vi "Find Optimal IRF Tail Slope.vi"(11 "Slope Array":dbl[](array[numeric])) -> (1 "Optimal Index":i32, 3 "Optimal Slope":dbl)   [LabVIEW 2021, in "Fits.lvlib"]
doc: "Find minimal absolute slope for the optimal IRF extraction algorithm."
uses:
  Fits.lvlib
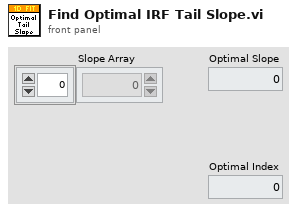
[diagram p1: front panel]
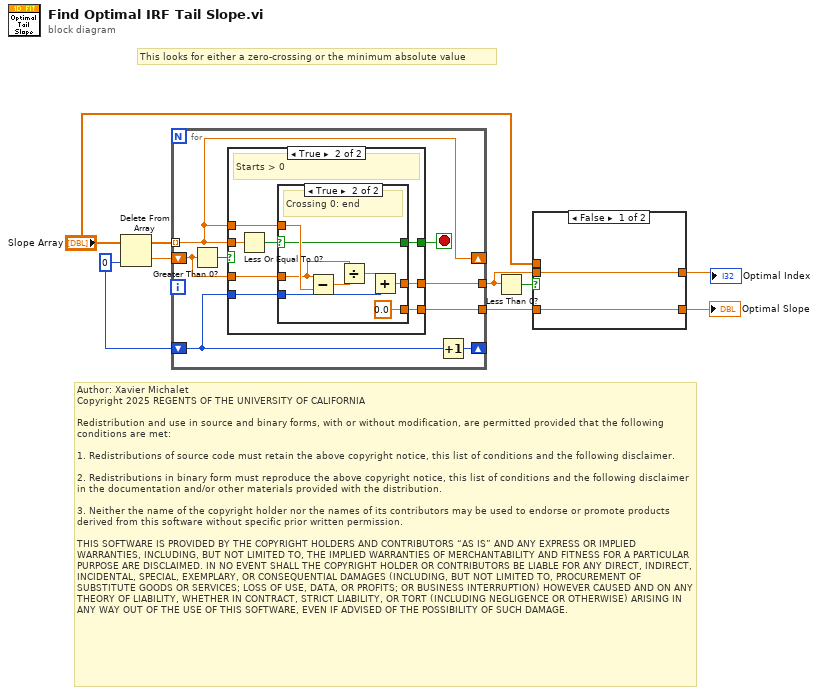
[diagram p0: block diagram]
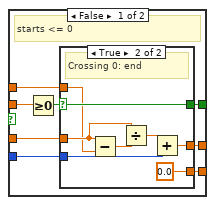
[diagram p2: hidden frame]
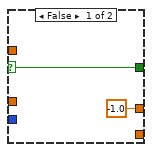
[diagram p3: hidden frame]
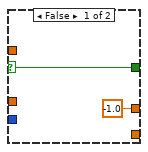
[diagram p4: hidden frame]
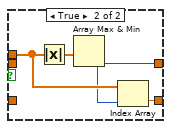
[diagram p5: hidden frame]
diagram:
  w7 = 0 ("index")
  # "Author: Xavier Michalet\nCopyright 2025 REGENTS OF THE UNIVERSITY OF CALIFORNIA\n\nRedistribution and use in source and binary forms, with or without modification, are permitted provided that the following conditions are met:\n\n1. Redistributions of source code must retain the above copyright notice, this list of conditions and the following disclaimer.\n\n2. Redistributions in binary form must reproduce the above copyright notice, this list of conditions and the following disclaimer in the documentation and/or other materials provided with the distribution.\n\n3. Neither the name of the copyright holder nor the names of its contributors may be used to endorse or promote products derived from this software without specific prior written permission.\n\nTHIS SOFTWARE IS PROVIDED BY THE COPYRIGHT HOLDERS AND CONTRIBUTORS “AS IS” AND ANY EXPRESS OR IMPLIED WARRANTIES, INCLUDING, BUT NOT LIMITED TO, THE IMPLIED WARRANTIES OF MERCHANTABILITY AND FITNESS FOR A PARTICULAR PURPOSE ARE DISCLAIMED. IN NO EVENT SHALL THE COPYRIGHT HOLDER OR CONTRIBUTORS BE LIABLE FOR ANY DIRECT, INDIRECT, INCIDENTAL, SPECIAL, EXEMPLARY, OR CONSEQUENTIAL DAMAGES (INCLUDING, BUT NOT LIMITED TO, PROCUREMENT OF SUBSTITUTE GOODS OR SERVICES; LOSS OF USE, DATA, OR PROFITS; OR BUSINESS INTERRUPTION) HOWEVER CAUSED AND ON ANY THEORY OF LIABILITY, WHETHER IN CONTRACT, STRICT LIABILITY, OR TORT (INCLUDING NEGLIGENCE OR OTHERWISE) ARISING IN ANY WAY OUT OF THE USE OF THIS SOFTWARE, EVEN IF ADVISED OF THE POSSIBILITY OF SUCH DAMAGE."
  # "This looks for either a zero-crossing or the minimum absolute value"
  n1 = Delete From Array(array="Slope Array", index=w7) -> (deleted portion=w9:dbl, array with subset deleted=w8:dbl[])  [unwired: 1 in]
  n2 = for {
    shift-right: [w12] -> _
    shift-left: w9 -> [w15]
    tunnel: w8 -> [w12] mode=indexing
    shift-right: [w16] -> _
    shift-left: w7 -> [w14]
    tunnel: [w13] -> w4
    tunnel: [w11] -> w2
    stop <- w10 stop-if-true
    n3 = Greater Than 0?(x=w15) -> (x > 0?=w17:bool)
    n4 = case shown="True" w17 {
      tunnel: w12 -> [w25 w43]
      tunnel: [w20 w37] -> w10
      tunnel: w12 -> [w23 w41]
      tunnel: w15 -> [w22 w40]
      tunnel: w14 -> [w21 w39]
      tunnel: [w19 w38] -> w13
      tunnel: [w18 w36] -> w11
      frame False {
        # "starts <= 0"
        n5 = Greater Or Equal To 0?(x=w25) -> (x >= 0?=w24:bool)
        n6 = case shown="True" w24 {
          selector: w24 -> [w27 w30]
          tunnel: w23 -> [_ w28]
          tunnel: w22 -> [_ w35]
          tunnel: w21 -> [_ w32]
          tunnel: [-1.0 w31] -> w19
          tunnel: [w27 w30] -> w20
          tunnel: [_ 0.0 ("Optimal Slope")] -> w18
          frame False {
          }
          frame True {
            # "Crossing 0: end"
            n7 = Subtract(x=w35, y=w28) -> (x-y=w34:dbl)
            n8 = Divide(x=w35, y=w34) -> (x/y=w33:dbl)
            n9 = Add(x=w33, y=w32) -> (x+y=w31:dbl)
          }
        }
      }
      frame True {
        # "Starts > 0"
        n10 = Less Or Equal To 0?(x=w43) -> (x <= 0?=w42:bool)
        n11 = case shown="True" w42 {
          selector: w42 -> [w45 w47]
          tunnel: w41 -> [_ w53]
          tunnel: w40 -> [_ w52]
          tunnel: w39 -> [_ w49]
          tunnel: [-1.0 w48] -> w38
          tunnel: [w45 w47] -> w37
          tunnel: [_ 0.0 ("Optimal Slope")] -> w36
          frame False {
          }
          frame True {
            # "Crossing 0: end"
            n12 = Subtract(x=w52, y=w53) -> (x-y=w51:dbl)
            n13 = Divide(x=w52, y=w51) -> (x/y=w50:dbl)
            n14 = Add(x=w50, y=w49) -> (x+y=w48:dbl)
          }
        }
      }
    }
    n15 = Increment(x=w14) -> (x+1=w16:i32)
  }
  n16 = Less Than 0?(x=w4) -> (x < 0?=w6:bool)
  n17 = case shown="False" w6 {
    tunnel: "Slope Array" -> [_ w58]
    tunnel: w4 -> [w55 _]
    tunnel: [w55 w56] -> w3
    tunnel: w2 -> [w54 _]
    tunnel: [w54 w57] -> w1
    frame False {
    }
    frame True {
      n18 = Absolute Value(x=w58) -> (abs(x)=w59:dbl[])
      n19 = Array Max & Min(array=w59) -> (min index (indices)=w56:i32)  [unwired: 3 out]
      n20 = Index Array(array=w58, index=w56) -> (element=w57:dbl)
    }
  }
  "Optimal Index" <- w3
  "Optimal Slope" <- w1
